vi "Acquire Sine Data.vi"(8 "Launch Order":i32, 9 "My Name":string) -> ()   [LabVIEW 2020, in "Startup Processes.lvlib"]
uses:
  Startup Processes.lvlib
  toolbox/Standard Signalling/ude_Stop Application/ude_Stop Application.lvlib
  toolbox/Standard Signalling/ude_Handle Errors/ude_Handle Errors.lvlib
  _buffers/Sample Rate/Sample Rate.lvlib
  _ude/Change Source/Change Source.lvlib
  _buffers/Plugin References/Plugin References.lvlib
  toolbox/User Interface/User Interface.lvlib
  Display Properties Manager/Display Properties Manager.lvlib
  _buffers/Sine Signal Data Buffer/Sine Signal Data Buffer.lvlib
  _buffers/Plugin Chart References/Plugin Chart References.lvlib
  _typedefs/Subpanel Names.ctl
  _ude/Read Graph Data/Read Graph Data.lvlib
panel:
  out "Acquired Data":dbl(graph)
  out "Error Out":errorcluster
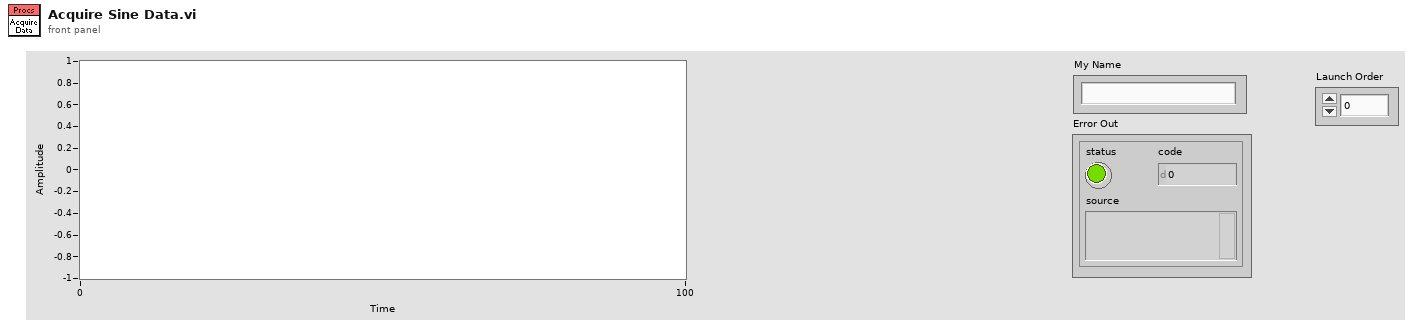
[diagram p1: front panel]
types:
  T1 = typedef "Startup Processes.lvlib/Subpanel Names.ctl" = enum16{"Sine Source", "Ramp Source", "Hen House TC", "Dog House TC", "Out House TC"}
  T2 = cluster{"reuse":refnum<event-registration>, "daq":refnum<event-registration>, "sys":refnum<event-registration>}
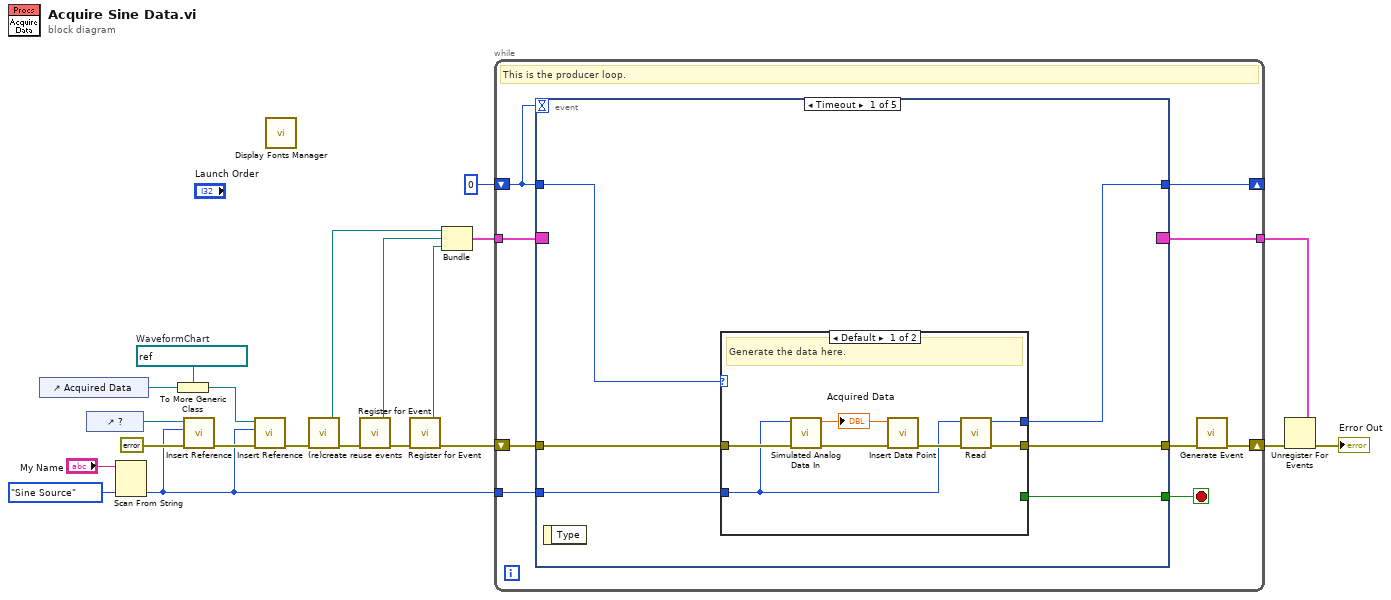
[diagram p0: block diagram]
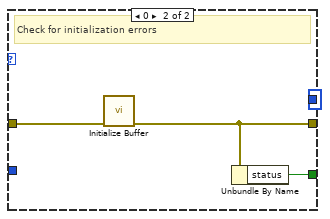
[diagram p2: hidden frame]
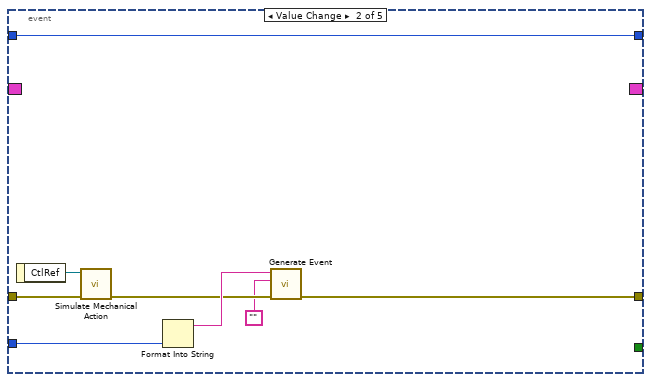
[diagram p3: hidden frame]
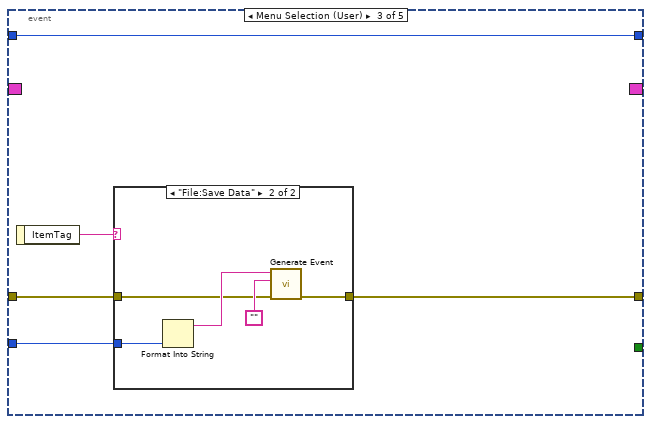
[diagram p4: hidden frame]
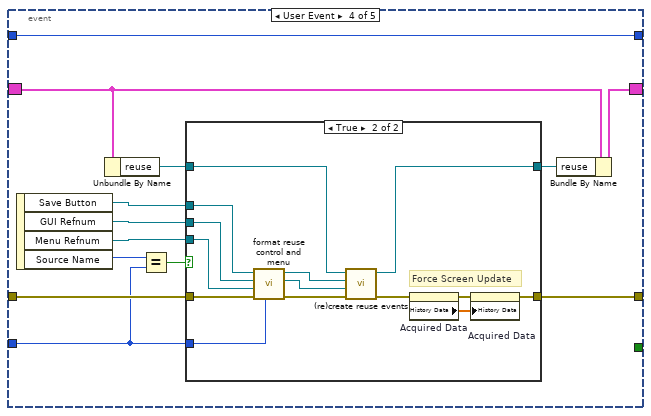
[diagram p6: hidden frame]
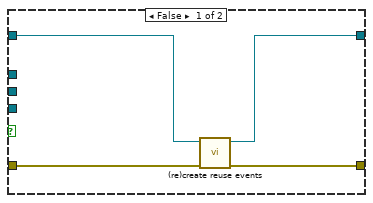
[diagram p7: hidden frame]
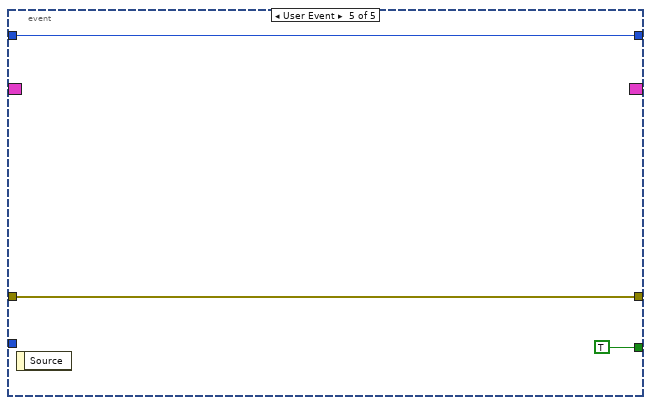
[diagram p8: hidden frame]
diagram:
  w7 = refnum<vi> refnum  # WaveformChart
  n1 = control-ref of="Acquired Data"() -> (w4:refnum<vi>)
  n2 = control-ref of="?"() -> (w11:refnum<vi>)
  n3 = Scan From String(input string="My Name", default 1=Subpanel_Names."Sine Source" ("Plugin Names")) -> (output 1=w1:T1)  [unwired: 3 in, 3 out]
  n4 = To More Generic Class(target class=w7, reference=w4) -> (generic class reference=w8:refnum<vi>)
  n5 = call "Insert Reference.vi"("Error In"=errorcluster {"status"=FALSE, "code"=0, "source"=""} ("Error Out"), "Plugin Name"=w1, "VI Refnum"=w11) -> ("Error Out"=w6:errorcluster)  [unwired: 4 in]
  n6 = call "Insert Reference.vi"("Error In"=w6, "Plugin Name"=w1, "WFChart Refnum"=w8) -> ("Error Out"=w5:errorcluster)  [unwired: 4 in]
  n7 = call "Display Fonts Manager.vi"() -> ()  [unwired: 7 in, 1 out]
  n8 = call "(re)create reuse events.vi"("error in (no error)"=w5) -> ("error out"=w9:errorcluster, "reuse"=w10:refnum<event-registration>)  [unwired: 5 in]
  n9 = call "Register for Event.vi"("Error In"=w9) -> ("Error Out"=w15:errorcluster, "daq"=w13:refnum<event-registration>)  [unwired: 5 in]
  n10 = call "Register for Event.vi"("Error In"=w15) -> ("Error Out"=w18:errorcluster, "sys"=w20:refnum<event-registration>)  [unwired: 5 in]
  n11 = Bundle("reuse"=w10, "daq"=w13, "sys"=w20) -> (w14:T2)  [unwired: 1 in]
  n12 = while {
    shift-right: [w26] -> w21
    shift-left: w18 -> [w30]
    tunnel: w14 -> [w29]
    tunnel: [w28] -> w19
    shift-right: [w23] -> _
    shift-left: 0 ("milliseconds to wait") -> [w24]
    tunnel: w1 -> [w22]
    stop <- w27 stop-if-true
    # "This is the producer loop."
    n13 = event shown="[0] Timeout" {
      selector: w29 -> [_ _ _ w72 _]
      dyn-events: [_ _ _ w73 _] -> w28
      timeout: w24 -> [_ _ _ _ _]
      tunnel: w30 -> [w36 w53 w57 w76 w100]
      tunnel: [w35 w49 w56 w75 w100] -> w25
      tunnel: [w32 _ _ _ TRUE] -> w27
      tunnel: w24 -> [w33 w55 w60 w79 w98]
      tunnel: [w34 w55 w60 w79 w98] -> w23
      tunnel: w22 -> [w31 w52 w58 w68 _]
      event Timeout {
        n14 = event-data() -> ()  [unwired: 1 in, 1 out]
        n15 = case shown="Default" w33 {
          tunnel: [w42 w44] -> w35
          tunnel: [w43 1 ("milliseconds to wait")] -> w34
          tunnel: [_ w46] -> w32
          tunnel: w36 -> [w41 w45]
          tunnel: w31 -> [w37 _]
          frame Default {
            # "Generate the data here."
            n16 = call "Simulated Analog Data In.vi"("error in (no error)"=w41, "Plugin Name"=w37) -> ("error out"=w39:errorcluster, "Simulated Data"=w40:dbl)  [unwired: 4 in]
            "Acquired Data" <- w40
            n17 = call "Insert Data Point.vi"("Error In"=w39, "Data"=w40) -> ("Error Out"=w38:errorcluster)  [unwired: 5 in]
            n18 = call "Read.vi"("Error In"=w38, "Plugin Name"=w37) -> ("Error Out"=w42:errorcluster, "Sample Period (msec)"=w43:i32)  [unwired: 4 in]
          }
          frame 0 {
            # "Check for initialization errors"
            n19 = call "Initialize Buffer.vi"("Error In"=w45) -> ("Error Out"=w44:errorcluster)  [unwired: 6 in]
            n20 = Unbundle By Name(w44) -> ("status"=w46:bool)
          }
        }
      }
      event Value Change {
        n21 = event-data() -> ("CtlRef"=w54:refnum<vi>)  [unwired: 1 in]
        n22 = call "Simulate Mechanical Action.vi"("Error In"=w53, "Button CtlRef"=w54) -> ("Error Out"=w50:errorcluster)  [unwired: 5 in]
        n23 = Format Into String(w52) -> (resulting string=w51:string)  [unwired: 3 in, 1 out]
        n24 = call "Generate Event.vi"("Error In"=w50, "Response Notifier"="", "Graph Name"=w51) -> ("Error Out"=w49:errorcluster)  [unwired: 4 in]
      }
      event Menu Selection (User) {
        n25 = event-data() -> ("ItemTag"=w59:string)  [unwired: 1 in]
        n26 = case shown="\"File:Save Data\"" w59 {
          tunnel: w58 -> [_ w63]
          tunnel: w57 -> [w61 w64]
          tunnel: [w61 w62] -> w56
          frame Default {
          }
          frame "File:Save Data" {
            n27 = Format Into String(w63) -> (resulting string=w66:string)  [unwired: 3 in, 1 out]
            n28 = call "Generate Event.vi"("Error In"=w64, "Response Notifier"="", "Graph Name"=w66) -> ("Error Out"=w62:errorcluster)  [unwired: 4 in]
          }
        }
      }
      event User Event {
        n29 = event-data() -> ("Save Button"=w71:refnum<vi>, "GUI Refnum"=w70:refnum<vi>, "Menu Refnum"=w69:refnum<k9>, "Source Name"=w67:T1)  [unwired: 1 in]
        n30 = Unbundle By Name(w72) -> ("reuse"=w77:refnum<event-registration>)
        n31 = Equal?(x=w67, y=w68) -> (x = y?=w74:bool)
        n32 = case shown="True" w74 {
          tunnel: w77 -> [w81 w97]
          tunnel: [w80 w96] -> w78
          tunnel: w76 -> [w83 w95]
          tunnel: [w82 w84] -> w75
          tunnel: w71 -> [_ w92]
          tunnel: w70 -> [_ w90]
          tunnel: w69 -> [_ w93]
          tunnel: w68 -> [_ w88]
          frame False {
            n33 = call "(re)create reuse events.vi"("error in (no error)"=w83, "reuse in"=w81) -> ("error out"=w82:errorcluster, "reuse"=w80:refnum<event-registration>)  [unwired: 4 in]
          }
          frame True {
            # "Force Screen Update"
            n34 = call "format reuse control and menu.vi"("My Name"=w88, "error in (no error)"=w95, "Menu Refnum"=w93, "GUI Refnum in"=w90, "Save Button"=w92) -> ("error out"=w94:errorcluster, "GUI Refnum out"=w89:refnum<vi>, "Save Button Out"=w91:refnum<vi>)  [unwired: 1 in]
            n35 = call "(re)create reuse events.vi"("error in (no error)"=w94, "Save Menu"=w89, "Save Button"=w91, "reuse in"=w97) -> ("error out"=w85:errorcluster, "reuse"=w96:refnum<event-registration>)  [unwired: 2 in]
            n36 = property on="Acquired Data" class="WFChart (strict)"(error in=w85) -> (error out=w86:errorcluster, "History Data"=w87:dbl[])  [unwired: 1 in, 1 out]
            n37 = property on="Acquired Data" class="WFChart (strict)"(error in=w86, "History Data"=w87) -> (error out=w84:errorcluster)  [unwired: 1 in, 1 out]
          }
        }
        n38 = Bundle By Name(cluster=w72, "reuse"=w78) -> (w73:T2)
      }
      event User Event {
        n39 = event-data() -> ()  [unwired: 1 in, 1 out]
      }
    }
    n40 = call "Generate Event.vi"("Error In"=w25) -> ("Error Out"=w26:errorcluster)  [unwired: 6 in]
  }
  n41 = Unregister For Events(event registration refnum=w19, error in=w21) -> (error out=→"Error Out":errorcluster)
